vi "Complete Service.vi"(0 "Room Service Monitor Model in":refnum<class "Room Service Monitor Model.lvclass">, 5 "Service ID":string, 11 "error in (no error)":errorcluster) -> (4 "Room Service Monitor Model out":refnum<class "Room Service Monitor Model.lvclass">, 15 "error out":errorcluster)   [LabVIEW 2023, in "Room Service Monitor Model.lvlib" / "Room Service Monitor Model.lvclass"]
uses:
  Room Service Monitor Model.lvclass
  Room Service Monitor Model.lvclass/Room Service Monitor Model.ctl
  <vilib>/ActorFramework/Actor/Actor.lvclass
  Interfaces/Incoming Hotel Management Tool Model Interface Messages/Update Service Completion Msg/Update Service Completion Msg.lvclass
  C:/Users/bhaghyaraj/Trainings/NI Actor Framework/SDLC/Model Base/Model Base/Model Base.lvclass
  C:/Program Files/National Instruments/LabVIEW 2023/vi.lib/ActorFramework/Actor/Actor.lvclass
  C:/Users/bhaghyaraj/Trainings/NI Actor Framework/SDLC/Interfaces/Model Base/Incoming Model Base Interface.lvclass
  C:/Users/bhaghyaraj/Trainings/NI Actor Framework/SDLC/Room Service Monitor Model/Room Service Monitor Model/Room Service Monitor Model.lvclass
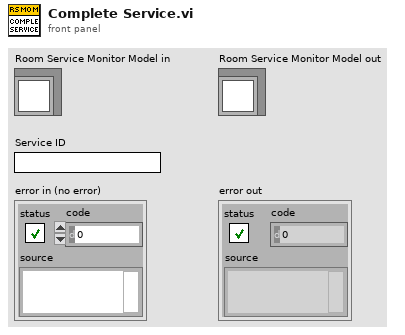
[diagram p1: front panel]
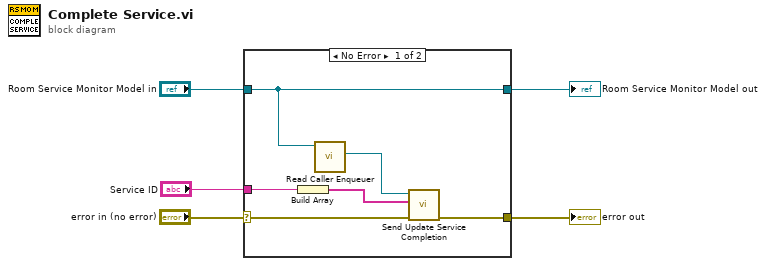
[diagram p0: block diagram]
diagram:
  n1 = case shown="No Error" "error in (no error)" {
    selector: "error in (no error)" -> [w11 w13]
    tunnel: [w10 w13] -> w4
    tunnel: [w9 w12] -> w2
    tunnel: "Room Service Monitor Model in" -> [w9 w12]
    tunnel: "Service ID" -> [w7 _]
    frame No Error {
      n2 = Build Array(w7) -> (w6:string[])
      n3 = call <vilib>:"Read Caller Enqueuer.vi"("Actor"=w9) -> ("Caller Enqueuer"=w8:refnum<class "Message Enqueuer.lvclass">)  [unwired: 10 in]
      n4 = call "Send Update Service Completion.vi"("error in (no error)"=w11, "Service ID"=w6, "Message Enqueuer"=w8) -> ("error out"=w10:errorcluster)  [unwired: 7 in, 1 out]
    }
    frame Error {
    }
  }
  "error out" <- w4
  "Room Service Monitor Model out" <- w2
